vi "ArcadeScaleLinear.vi"(10 "Direction":dbl format="%#_13g") -> (2 "Scale":dbl)   [LabVIEW 2013]
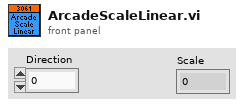
[diagram p1: front panel]
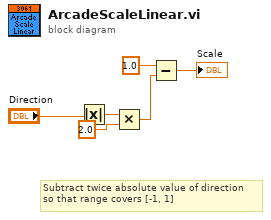
[diagram p0: block diagram]
diagram:
  # "Subtract twice absolute value of direction\nso that range covers [-1, 1]"
  n1 = Absolute Value(x="Direction") -> (abs(x)=w5:dbl)
  n2 = Multiply(x=w5, y=2.0) -> (x*y=w3:dbl)
  n3 = Subtract(x=1.0, y=w3) -> (x-y=→"Scale":dbl)
